vi "uTTA_GetPGAGain.vi"(8 "error in":errorcluster, 11 "VISA Refnum in":refnum<visa-resource-name>) -> (0 "error out":errorcluster, 3 "VISA Refnum out":refnum<visa-resource-name>, 4 "PGA Gain(ms)":u32, 7 "Received":string)   [LabVIEW 2021]
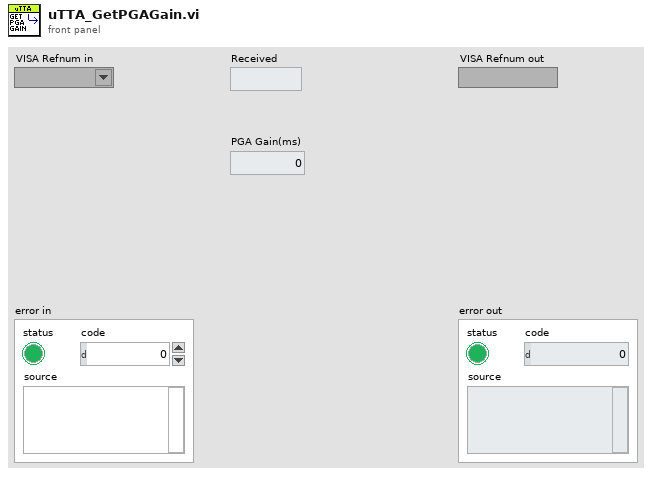
[diagram p1: front panel]
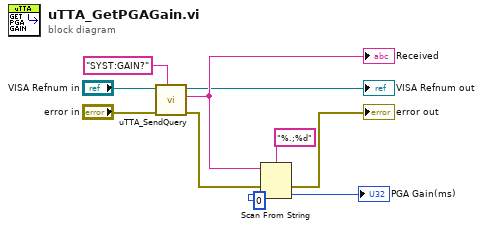
[diagram p0: block diagram]
diagram:
  n1 = call "uTTA_SendQuery.vi"("Send String"="SYST:GAIN?" ("format string"), "error in (no error)"="error in", "VISA Refnum in"="VISA Refnum in") -> ("error out"=w8:errorcluster, "Received"=w6:string, "VISA Refnum out"=→"VISA Refnum out":refnum<visa-resource-name>)  [unwired: 6 in]
  "Received" <- w6
  n2 = Scan From String(format string="%.;%d", input string=w6, error in=w8, default 1=u32 0 ("default value 1")) -> (error out=→"error out":errorcluster, output 1=→"PGA Gain(ms)":u32)  [unwired: 1 in, 2 out]
